vi "Get SLSC Module By Name.vi"(8 "error in (no error)":errorcluster, 10 "Name":string, 11 "SLSC Chassis":u64) -> (0 "error out":errorcluster, 1 "Found":bool, 2 "SLSC Module":u64, 3 "SLSC Chassis out":u64)   [LabVIEW 2020, in "VeriStand SLSC Scripting.lvlib"]
uses:
  VeriStand SLSC Scripting.lvlib
  NationalInstruments.VeriStand.SystemDefinitionAPI
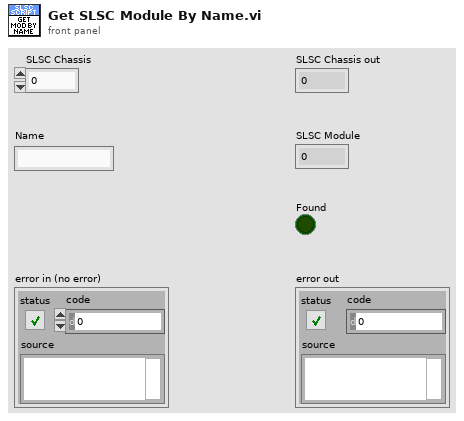
[diagram p1: front panel]
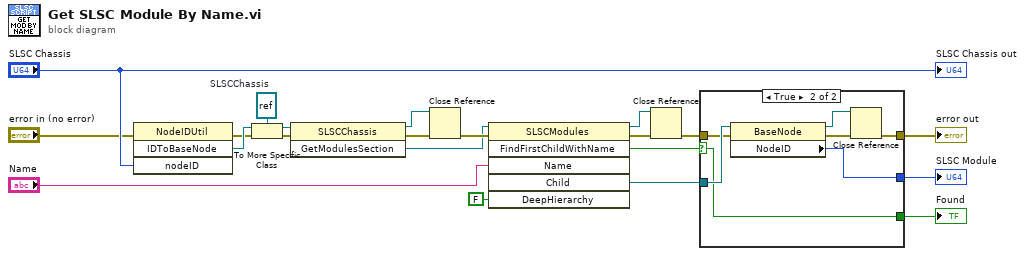
[diagram p0: block diagram]
diagram:
  w6 = refnum<k24> refnum  # SLSCChassis
  n1 = invoke class="NodeIDUtil" method="IDToBaseNode"(error in="error in (no error)", "nodeID"="SLSC Chassis") -> (error out=w5:errorcluster, "IDToBaseNode"=w7:refnum<k24>)  [unwired: 2 in, 2 out]
  n2 = To More Specific Class(target class=w6, reference=w7, error in=w5) -> (specific class reference=w3:refnum<k24>, error out=w4:errorcluster)
  n3 = invoke class="SLSCChassis" method="GetModulesSection"(reference=w3, error in=w4) -> (reference out=w2:refnum<k24>, error out=w9:errorcluster, "GetModulesSection"=w1:refnum<k24>)  [unwired: 1 in]
  n4 = Close Reference(reference=w2, error in (no error)=w9) -> (error out=w8:errorcluster)
  n5 = invoke class="SLSCModules" method="FindFirstChildWithName"(reference=w1, error in=w8, "Name"="Name", "DeepHierarchy"=FALSE) -> (reference out=w13:refnum<k24>, error out=w16:errorcluster, "FindFirstChildWithName"=w12:bool, "Child"=w15:refnum<k24>)  [unwired: 2 in, 2 out]
  n6 = Close Reference(reference=w13, error in (no error)=w16) -> (error out=w14:errorcluster)
  n7 = case shown="True" w12 {
    selector: w12 -> [w22 w27]
    tunnel: [w23 w25] -> w10
    tunnel: [_ w30] -> w19
    tunnel: w15 -> [_ w29]
    tunnel: w14 -> [w23 w28]
    tunnel: [w22 w27] -> w11
    frame False {
    }
    frame True {
      n8 = property class="BaseNode"(reference=w29, error in=w28) -> (reference out=w24:refnum<k24>, error out=w26:errorcluster, "NodeID"=w30:u64)
      n9 = Close Reference(reference=w24, error in (no error)=w26) -> (error out=w25:errorcluster)
    }
  }
  "error out" <- w10
  "SLSC Module" <- w19
  "Found" <- w11
  "SLSC Chassis out" <- "SLSC Chassis"
